vi "Time Info To Format String.vi"(11 "Time Format & Precision Info":T1) -> (3 "Format String":string)   [LabVIEW 2018, in "Numeric Data Type.lvclass"]
uses:
  Numeric Data Type.lvclass
  Time Info.ctl
  Time Format.ctl
  Numeric Format Enum.ctl
  Clock Type.ctl
  Date Order.ctl
  Date Format.ctl
  Year Format.ctl
panel:
  in  "Date Separator":string="/"
  in  "Time Separator":string=":"
  # "(10 = Absolute)"
  # "0 = Local (No DST String)\n1 = UTC (No DST String)\n2 = Local (With DST String)\n3 = UTC (With DST String)"
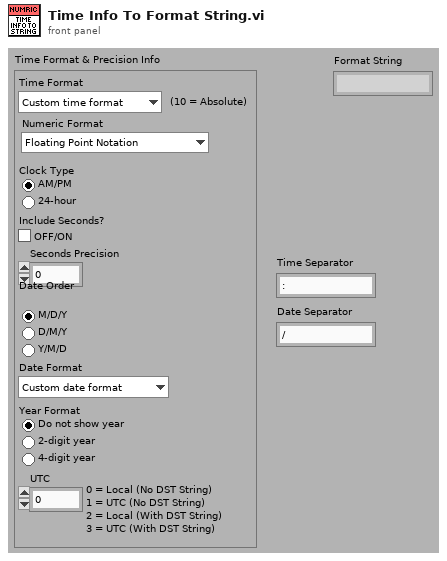
[diagram p1: front panel]
types:
  T1 = typedef "Numeric Data Type.lvclass/Time Info.ctl" = cluster{"Time Format":T2, "Numeric Format":T3, "Clock Type":T4, "Include Seconds?":bool, "Seconds Precision":i16, "Date Order":T5, "Date Format":T6, "Year Format":T7, "UTC":i16}
  T2 = typedef "Numeric Data Type.lvclass/Time Format.ctl" = enum16{"Custom time format", "System time format", "Time unused"}
  T3 = typedef "Numeric Data Type.lvclass/Numeric Format Enum.ctl" = enum16{"Floating Point Notation", "Scientific Notation", "Engineering Notation", "SI Notation", "<not used>", "Decimal", "Hexadecimal", "Octal", "Binary", "<not used 2>", "Absolute Time", "Relative Time"}
  T4 = typedef "Numeric Data Type.lvclass/Clock Type.ctl" = enum32{"12-Hour (AM/PM)", "24-Hour"}
  T5 = typedef "Numeric Data Type.lvclass/Date Order.ctl" = enum32{"M/D/Y", "D/M/Y", "Y/M/D"}
  T6 = typedef "Numeric Data Type.lvclass/Date Format.ctl" = enum16{"Custom date format", "System date format", "Date unused"}
  T7 = typedef "Numeric Data Type.lvclass/Year Format.ctl" = enum32{"No Year", "2-digit Year", "4-digit Year"}
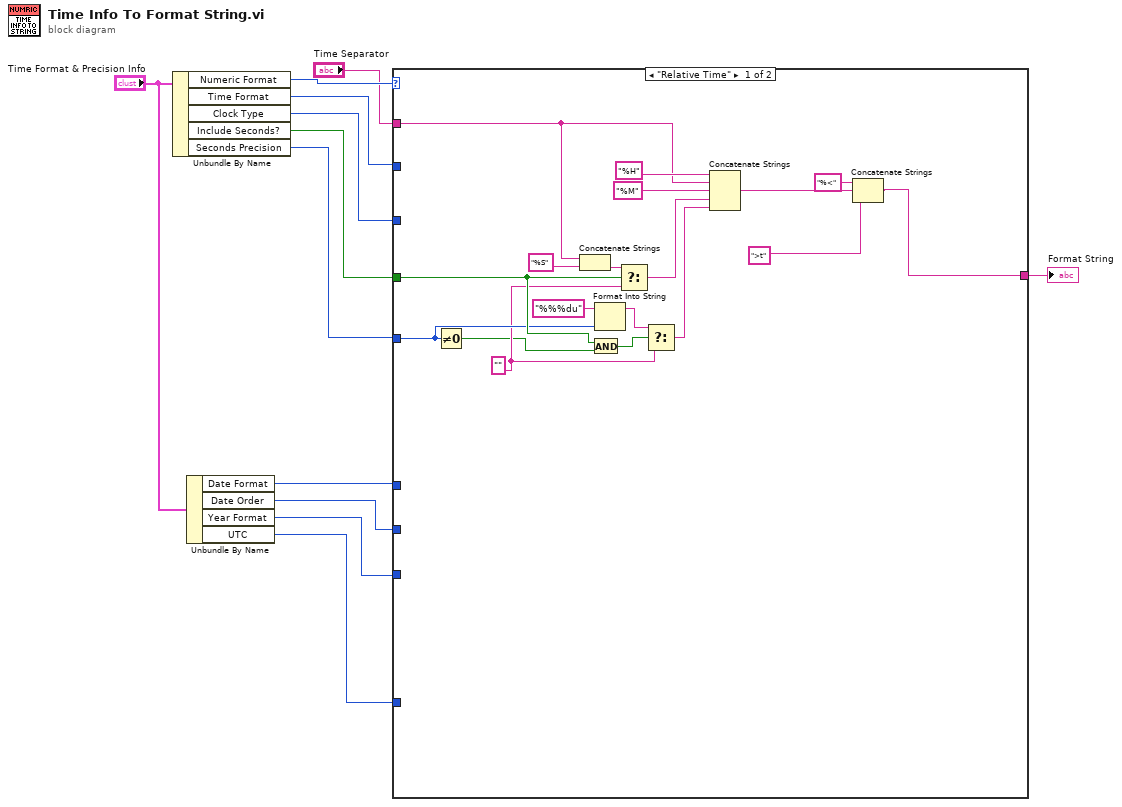
[diagram p0: block diagram]
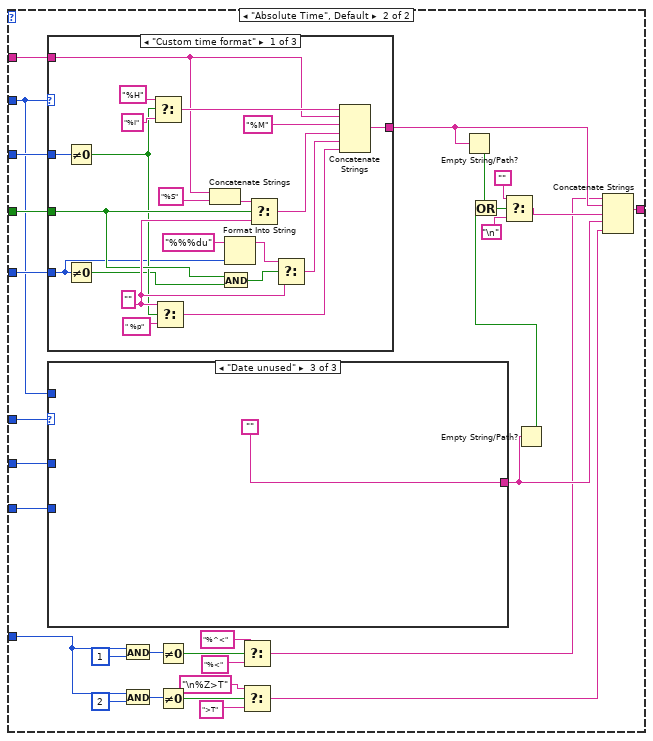
[diagram p2: hidden frame]
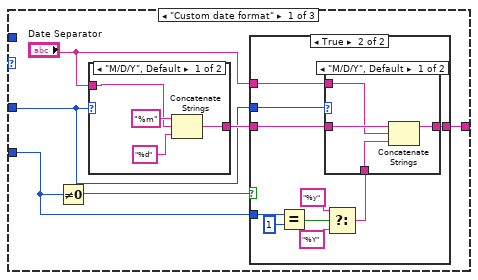
[diagram p3: hidden frame]
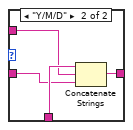
[diagram p5: hidden frame]
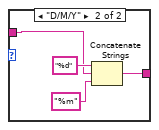
[diagram p6: hidden frame]
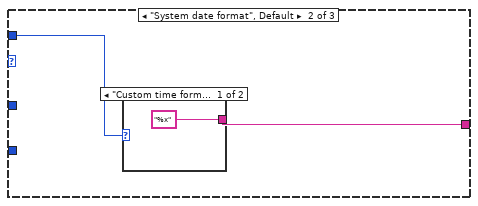
[diagram p7: hidden frame]
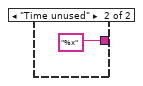
[diagram p8: hidden frame]
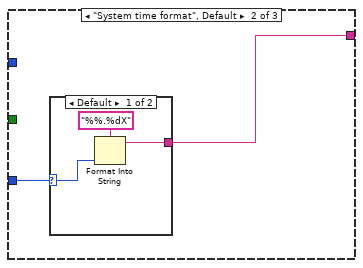
[diagram p9: hidden frame]
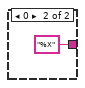
[diagram p10: hidden frame]
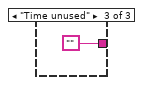
[diagram p11: hidden frame]
diagram:
  n1 = Unbundle By Name("Time Format & Precision Info") -> ("Numeric Format"=w12:T3, "Time Format"=w10:T2, "Clock Type"=w9:T4, "Include Seconds?"=w8:bool, "Seconds Precision"=w7:i16)
  n2 = Unbundle By Name("Time Format & Precision Info") -> ("Date Format"=w6:T6, "Date Order"=w5:T5, "Year Format"=w4:T7, "UTC"=w3:i16)
  n3 = case shown="\"Relative Time\"" w12 {
    tunnel: w6 -> [_ w60]
    tunnel: w9 -> [_ w59]
    tunnel: w8 -> [w30 w58]
    tunnel: w7 -> [w29 w57]
    tunnel: w5 -> [_ w56]
    tunnel: w4 -> [_ w55]
    tunnel: [w26 w54] -> w1
    tunnel: w10 -> [_ w53]
    tunnel: "Time Separator" -> [w14 w52]
    tunnel: w3 -> [_ w34]
    frame "Relative Time" {
      w21 = ""
      n4 = Not Equal To 0?(x=w29) -> (x != 0?=w16:bool)
      n5 = Concatenate Strings(w14, "%S") -> (w24:string)
      n6 = And(x=w30, y=w16) -> (x .and. y?=w17:bool)
      n7 = Format Into String(format string="%%%du", w29) -> (resulting string=w20:string)  [unwired: 2 in, 1 out]
      n8 = Select(t=w24, s=w30, f=w21) -> (s? t:f=w22:string)
      n9 = Select(t=w20, s=w17, f=w21) -> (s? t:f=w19:string)
      n10 = Concatenate Strings("%H", w14, "%M" ("string"), w22, w19) -> (w28:string)
      n11 = Concatenate Strings("%<" ("string"), w28, ">t") -> (w26:string)
    }
    frame "Absolute Time", Default {
      n12 = case shown="\"Custom time format\"" w53 {
        tunnel: [w111 w120 ""] -> w51
        tunnel: w59 -> [w103 _ _]
        tunnel: w58 -> [w104 _ _]
        tunnel: w57 -> [w101 w121 _]
        tunnel: w52 -> [w99 _ _]
        frame "Custom time format" {
          w110 = ""
          n13 = Not Equal To 0?(x=w103) -> (x != 0?=w102:bool)
          n14 = Not Equal To 0?(x=w101) -> (x != 0?=w100:bool)
          n15 = Select(t="%H", s=w102, f="%I") -> (s? t:f=w116:string)
          n16 = Select(t=w110, s=w102, f=" %p") -> (s? t:f=w106:string)
          n17 = Concatenate Strings(w99, "%S") -> (w114:string)
          n18 = And(x=w104, y=w100) -> (x .and. y?=w105:bool)
          n19 = Format Into String(format string="%%%du", w101) -> (resulting string=w109:string)  [unwired: 2 in, 1 out]
          n20 = Select(t=w114, s=w104, f=w110) -> (s? t:f=w112:string)
          n21 = Select(t=w109, s=w105, f=w110) -> (s? t:f=w108:string)
          n22 = Concatenate Strings(w116, w99, "%M" ("string"), w112, w108, w106) -> (w111:string)
        }
        frame "System time format", Default {
          n23 = case shown="Default" w121 {
            selector: w121 -> [w124 _]
            tunnel: [w123 "%X"] -> w120
            frame Default {
              n24 = Format Into String(format string="%%.%dX", w124) -> (resulting string=w123:string)  [unwired: 2 in, 1 out]
            }
            frame 0 {
            }
          }
        }
        frame "Time unused" {
        }
      }
      n25 = case shown="\"Date unused\"" w60 {
        tunnel: [w62 w95 ""] -> w45
        tunnel: w56 -> [w65 _ _]
        tunnel: w55 -> [w63 _ _]
        tunnel: w53 -> [_ w94 _]
        frame "Custom date format" {
          n26 = Not Equal To 0?(x=w63) -> (x != 0?=w64:bool)
          n27 = case shown="\"M/D/Y\", Default" w65 {
            tunnel: "Date Separator" -> [w88 w92]
            tunnel: [w86 w90] -> w66
            frame "M/D/Y", Default {
              n28 = Concatenate Strings("%m", w88, "%d") -> (w86:string)
            }
            frame "D/M/Y" {
              n29 = Concatenate Strings("%d", w92, "%m") -> (w90:string)
            }
          }
          n30 = case shown="True" w64 {
            tunnel: w66 -> [w67 w77]
            tunnel: "Date Separator" -> [_ w76]
            tunnel: w65 -> [_ w75]
            tunnel: w63 -> [_ w71]
            tunnel: [w67 w68] -> w62
            frame False {
            }
            frame True {
              n31 = Equal?(x=w71, y=i16 1) -> (x = y?=w72:bool)
              n32 = Select(t="%y", s=w72, f="%Y") -> (s? t:f=w69:string)
              n33 = case shown="\"M/D/Y\", Default" w75 {
                tunnel: w77 -> [w81 w82]
                tunnel: w76 -> [w78 w83]
                tunnel: w69 -> [w80 w84]
                tunnel: [w79 w85] -> w68
                frame "M/D/Y", Default {
                  n34 = Concatenate Strings(w81, w78, w80) -> (w79:string)
                }
                frame "Y/M/D" {
                  n35 = Concatenate Strings(w84, w83, w82) -> (w85:string)
                }
              }
            }
          }
        }
        frame "System date format", Default {
          n36 = case shown="\"Custom time format\", Default" w94 {
            tunnel: ["%x" "%x"] -> w95
            frame "Custom time format", Default {
            }
            frame "Time unused" {
            }
          }
        }
        frame "Date unused" {
        }
      }
      n37 = And(x=w34, y=i16 1) -> (x .and. y?=w40:i16)
      n38 = And(x=w34, y=i16 2) -> (x .and. y?=w37:i16)
      n39 = Not Equal To 0?(x=w40) -> (x != 0?=w39:bool)
      n40 = Not Equal To 0?(x=w37) -> (x != 0?=w38:bool)
      n41 = Select(t="%^<", s=w39, f="%<") -> (s? t:f=w33:string)
      n42 = Select(t="\n%Z>T", s=w38, f=">T") -> (s? t:f=w32:string)
      n43 = Empty String/Path?(string/path=w51) -> (empty?=w50:bool)
      n44 = Empty String/Path?(string/path=w45) -> (empty?=w49:bool)
      n45 = Or(x=w50, y=w49) -> (x .or. y?=w48:bool)
      n46 = Select(t="", s=w48, f="\n") -> (s? t:f=w44:string)
      n47 = Concatenate Strings(w33, w51, w44, w45, w32) -> (w54:string)
    }
  }
  "Format String" <- w1
